vi "MaxTime.vi"(1 "MaxTime":dbl, 2 "Reset?":bool) -> (0 "Finished?":bool)   [LabVIEW 2015]
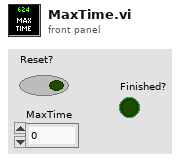
[diagram p1: front panel]
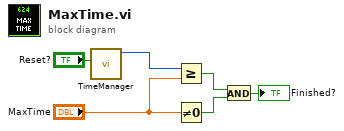
[diagram p0: block diagram]
diagram:
  n1 = call "TimeManager.vi"("Reset?"="Reset?") -> ("Time Since Reset"=w4:u32)  [unwired: 9 in, 1 out]
  n2 = Greater Or Equal?(x=w4, y="MaxTime") -> (x >= y?=w3:bool)
  n3 = Not Equal To 0?(x="MaxTime") -> (x != 0?=w2:bool)
  n4 = And(x=w3, y=w2) -> (x .and. y?=→"Finished?":bool)
